vi "New ADS1X15 Device.vi"(8 "error in (no error)":errorcluster, 9 "ADC Type (ADS1015)":T1, 10 "I2C Slave Address (0x48)":u8=72 format="%.0x", 11 "I2C":refnum<class "LINX I2C.lvclass">) -> (0 "error out":errorcluster, 3 "LINX-ADS1X15 out":refnum<class "LINX-ADS1X15.lvclass">)   [LabVIEW 2020, in "LINX-ADS1X15.lvclass"]
uses:
  LINX-ADS1X15.lvclass
  LINX I2C/LINX I2C.lvclass
  ADC Type Selection.ctl
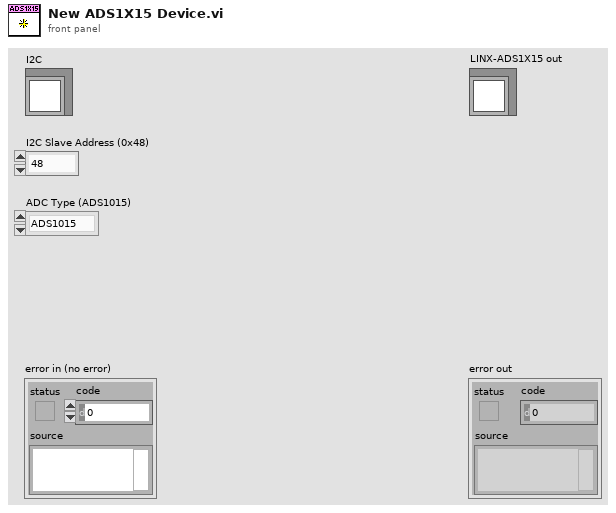
[diagram p1: front panel]
types:
  T1 = typedef "LINX-ADS1X15.lvclass/ADC Type Selection.ctl" = enum16{"ADS1015", "ADS1115"}
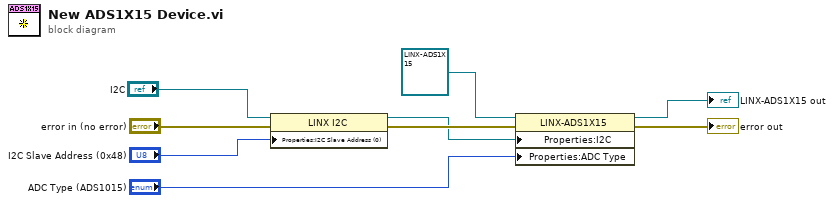
[diagram p0: block diagram]
diagram:
  n1 = property class="LINX I2C"(reference="I2C", error in="error in (no error)", "Properties:I2C Slave Address (0)"="I2C Slave Address (0x48)") -> (reference out=w6:refnum<class "LINX I2C.lvclass">, error out=w7:errorcluster)
  n2 = property class="LINX-ADS1X15"(reference=refnum<class "LINX-ADS1X15.lvclass"> refnum ("LINX-ADS1X15 in"), error in=w7, "Properties:I2C"=w6, "Properties:ADC Type"="ADC Type (ADS1015)") -> (reference out=→"LINX-ADS1X15 out":refnum<class "LINX-ADS1X15.lvclass">, error out=→"error out":errorcluster)
